vi "Read Dual Part.vi"(11 "Dual in":refnum<class "Dual.lvclass">) -> (1 "Dual Part":dbl, 3 "Dual out":refnum<class "Dual.lvclass">)   [LabVIEW 2020, in "Automatic Differentiation.lvlib" / "Dual.lvclass"]
uses:
  Dual.lvclass
  Dual.lvclass/Dual.ctl
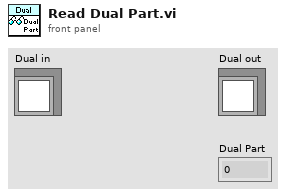
[diagram p1: front panel]
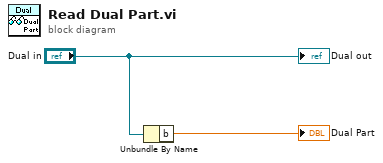
[diagram p0: block diagram]
diagram:
  n1 = Unbundle By Name("Dual in") -> ("b"=→"Dual Part":dbl)
  "Dual out" <- "Dual in"
